vi "Create Dir if Non-Existant__ogtk.vi"(8 "error in (no error)":errorcluster, 9 "permissions (0755)":i16=493 format="%.0o", 11 "Directory Path":path) -> (0 "error out":errorcluster, 2 "Created Directories":path[](array[path]), 3 "dup Directory Path":path)   [LabVIEW 2020]
doc: "Will create all directories above and including the directory defined by the \"Directory Path\" input, if they do not already exist."
panel:
  # "Create Dir if Non-Existant.vi\n\nWill create all directories above and including the directory defined by the \"Directory Path\" input, if they do not already exist.\n\nPlease visit http://www.OpenG.org to learn about the\nOpen Source LabVIEW software movement.\n\nNOTICE -- YOU MUST LEAVE THIS NOTICE IN PLACE.  PER THE TERMS OF THE LICENSE BELOW, YOU MAY SUBLICENSE THIS SOFTWARE \nIN ANY WAY THAT DOES NOT CONFLICT WITH THIS LICENSE.\n\n### BSD License (http://www.opensource.org/licenses/bsd-license.php) Begin ###\n \nCopyright (c) 2002-2006, Jim Kring <jim@jimkring.com>\nCopyright (c) 2002, Cal-Bay Systems, Inc. <info@calbay.com>\n\nAll rights reserved.\n\nRedistribution and use in source and binary forms, with or without modification, are permitted provided that the following conditions are met:\n\n    * Redistributions of source code must retain the above copyright notice, this list of conditions and the following disclaimer.\n    * Redistributions in binary form must reproduce the above copyright notice, this list of conditions and the following disclaimer in the \n       documentation and/or other materials provided with the distribution.\n    * Neither the name of SciWare, James Kring, Inc., nor the names of its contributors may be used to endorse or promote products derived \n       from this software without specific prior written permission.\n\nTHIS SOFTWARE IS PROVIDED BY THE COPYRIGHT HOLDERS AND CONTRIBUTORS \"AS IS\" AND ANY EXPRESS OR IMPLIED WARRANTIES, \nINCLUDING, BUT NOT LIMITED TO, THE IMPLIED WARRANTIES OF MERCHANTABILITY AND FITNESS FOR A PARTICULAR PURPOSE ARE \nDISCLAIMED. IN NO EVENT SHALL THE COPYRIGHT OWNER OR CONTRIBUTORS BE LIABLE FOR ANY DIRECT, INDIRECT, INCIDENTAL,\n SPECIAL, EXEMPLARY, OR CONSEQUENTIAL DAMAGES (INCLUDING, BUT NOT LIMITED TO, PROCUREMENT OF SUBSTITUTE GOODS OR \nSERVICES; LOSS OF USE, DATA, OR PROFITS; OR BUSINESS INTERRUPTION) HOWEVER CAUSED AND ON ANY THEORY OF LIABILITY, \nWHETHER IN CONTRACT, STRICT LIABILITY, OR TORT (INCLUDING NEGLIGENCE OR OTHERWISE) ARISING IN ANY WAY OUT OF THE USE \nOF THIS SOFTWARE, EVEN IF ADVISED OF THE POSSIBILITY OF SUCH DAMAGE.\n\n### BSD License End ###"
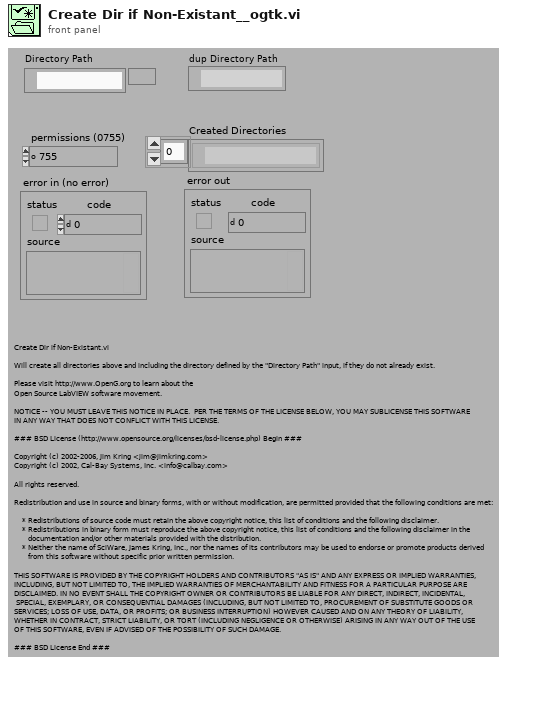
[diagram p1: front panel]
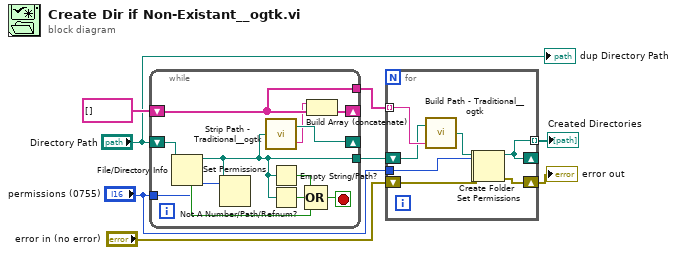
[diagram p0: block diagram]
diagram:
  n1 = while {
    shift-right: [w12] -> _
    shift-left: "Directory Path" -> [w19]
    shift-right: [w18] -> _
    shift-left: string[] [] -> [w17]
    tunnel: [w17] -> w5
    tunnel: [w10] -> w4
    tunnel: "permissions (0755)" -> [w9]
    stop <- w16 stop-if-true
    n2 = File/Directory Info(path=w19) -> (path out=w10:path, directory=w13:bool)  [unwired: 1 in, 5 out]
    n3 = Set Permissions(7:w9, 11:w10) -> ()  [unwired: 3 in, 2 out]
    n4 = call <userlib>:"Strip Path - Traditional__ogtk.vi"("path"=w10) -> ("stripped path"=w12:path, "name"=w11:string)
    n5 = Empty String/Path?(string/path=w10) -> (empty?=w15:bool)
    n6 = Not A Number/Path/Refnum?(number/path/refnum=w10) -> (NaN/Path/Refnum?=w14:bool)
    n7 = Compound Arithmetic op=OR(w15, w14, w13) -> (w16:bool)
    n8 = Build Array (concatenate)(w11, w17) -> (w18:string[])
  }
  n9 = for {
    tunnel: w5 -> [w28] mode=indexing
    shift-right: [w22] -> _
    shift-left: w4 -> [w27]
    shift-right: [w26] -> w7
    shift-left: "error in (no error)" -> [w25]
    tunnel: "permissions (0755)" -> [w23]
    tunnel: [w22] -> w1 mode=indexing
    n10 = call <userlib>:"Build Path - Traditional__ogtk.vi"("name or relative path"=w28, "base path"=w27) -> ("appended path"=w24:path)
    n11 = Create Folder(path (use dialog)=w24, error in=w25) -> (created path=w21:path, error out=w20:errorcluster)  [unwired: 1 in, 1 out]
    n12 = Set Permissions(7:w23, 8:w20, 11:w21) -> (0:w26:errorcluster, 3:w22:path)  [unwired: 2 in]
  }
  "error out" <- w7
  "Created Directories" <- w1
  "dup Directory Path" <- "Directory Path"
